vi "UTIL Save Raw Data.vi"(6 "Testing":bool, 8 "Error In":errorcluster, 11 "EMG and EEG":waveform(dbl)[](array[waveform])) -> (0 "Error Out":errorcluster, 3 "Hourly File Path":path)   [LabVIEW 2010]
doc: "This VI saves the raw EMG and EEG Samples to a data file. At present, a new data file is created every hour, having the date and time recorded as part of the file name. Every time this VI is called, it opens the appropriate file, goes to the end of the file, writes the data, and closes the file, thus guarding against a crash in the middle of a recording session.\n\nIf there are no data to save, we just return the current Hourly File Path.\n\nA Testing input allows choosing to save the files in the LabVIEW Temp directory.\n\nInputs:\n EMG and EEG Array of Analog Sampling Waveforms\n Testing Boolean (default False), selects Temp directory if True\n Error In\nOutputs:\n Hourly File Path Last-named Output File Path\n Error Out"
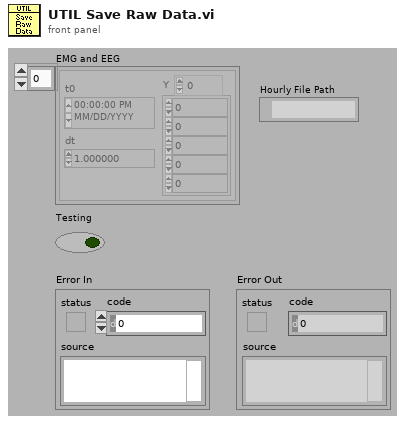
[diagram p1: front panel]
types:
  T1 = enum16{"open", "replace", "create", "open or create", "replace or create", "replace or create with confirmation"}
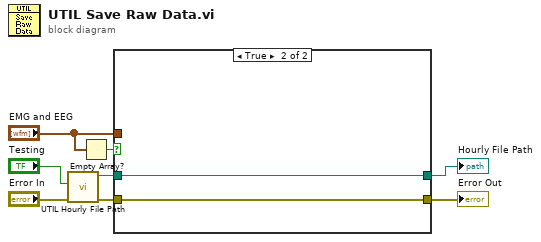
[diagram p0: block diagram]
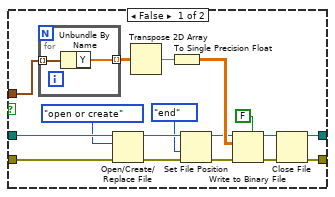
[diagram p2: hidden frame]
diagram:
  n1 = call "UTIL Hourly File Path.vi"("Error In"="Error In", "Testing"="Testing") -> ("Error Out"=w7:errorcluster, "Hourly File Path"=w5:path)  [unwired: 8 in]
  n2 = Empty Array?(array="EMG and EEG") -> (empty?=w2:bool)
  n3 = case shown="True" w2 {
    tunnel: w7 -> [w25 w28]
    tunnel: w5 -> [w24 w29]
    tunnel: "EMG and EEG" -> [w23 _]
    tunnel: [w10 w28] -> w4
    tunnel: [w9 w29] -> w3
    frame False {
      n4 = for {
        tunnel: w23 -> [w27] mode=indexing
        tunnel: [w26] -> w12 mode=indexing
        n5 = Unbundle By Name(w27) -> ("Y"=w26:dbl[])
      }
      n6 = Open/Create/Replace File(file path (use dialog)=w24, error in=w25, operation (0:open)=T1."open or create") -> (refnum out=w16:refnum<file>, error out=w17:errorcluster)  [unwired: 3 in, 1 out]
      n7 = Transpose 2D Array(2D array=w12) -> (transposed array=w22:dbl[][])
      n8 = To Single Precision Float(number=w22) -> (single precision float=w19:sgl[][])
      n9 = Set File Position(refnum=w16, from (0:start)=enum16{"start", "end", "current"}."end", error in=w17) -> (refnum out=w14:refnum<file>, error out=w13:errorcluster)  [unwired: 1 in]
      n10 = Write to Binary File(file (use dialog)=w14, data=w19, error in=w13, 5:FALSE ("prepend array or string size? (T)")) -> (refnum out=w11:refnum<file>, error out=w18:errorcluster)  [unwired: 2 in, 1 out]
      n11 = Close File(refnum=w11, error in=w18) -> (path=w9:path, error out=w10:errorcluster)
    }
    frame True {
    }
  }
  "Error Out" <- w4
  "Hourly File Path" <- w3
